vi "Update.vi"(8 "error in":errorcluster, 11 "Data Subject in":refnum<class "Data Subject.lvclass">) -> (0 "error out":errorcluster, 2 "Stop?":bool, 3 "Data Subject out":refnum<class "Data Subject.lvclass">)   [LabVIEW 2015, in "Data Subject.lvclass"]
doc: "Default action of the Update function is strictly to see if a stop execution has been sent."
uses:
  Data Subject.lvclass
  Data Subject.lvclass/Data Subject.ctl
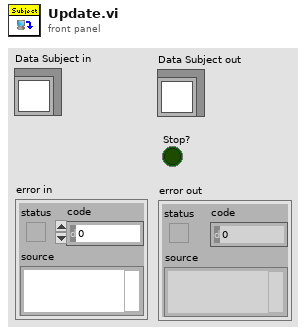
[diagram p1: front panel]
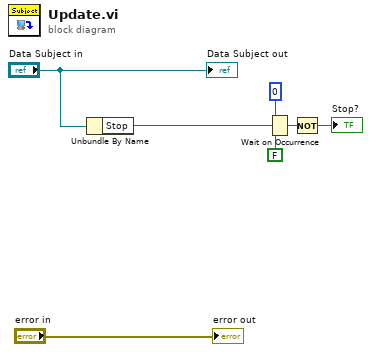
[diagram p0: block diagram]
diagram:
  n1 = Unbundle By Name("Data Subject in") -> ("Stop"=w4:refnum<k4>)
  n2 = Wait on Occurrence(1:FALSE ("ignore previous (T)"), 2:w4, 3:0 ("ms timeout (-1)")) -> (0:w1:bool)
  n3 = Not(x=w1) -> (.not. x?=→"Stop?":bool)
  "error out" <- "error in"
  "Data Subject out" <- "Data Subject in"
